vi "hmi_browse_builder_class.vi"(8 "error in (no error)":errorcluster, 11 "project_file":string) -> (0 "error out":errorcluster, 3 "selected path":path)   [LabVIEW 2015, in "lv-build-interface.lvlib"]
uses:
  lv-build-interface.lvlib
  lv-builder/lv-builder.lvlib
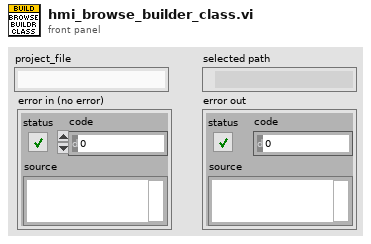
[diagram p1: front panel]
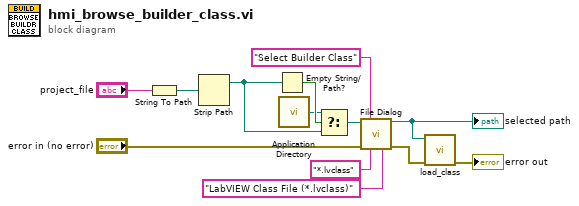
[diagram p0: block diagram]
diagram:
  n1 = String To Path(string="project_file") -> (path=w11:path)
  n2 = Strip Path(path=w11) -> (stripped path=w4:path)  [unwired: 1 out]
  n3 = Empty String/Path?(string/path=w4) -> (empty?=w12:bool)
  n4 = call <vilib>:"Application Directory.vi"() -> ("Application Directory"=w9:path)
  n5 = Select(t=w9, s=w12, f=w4) -> (s? t:f=w13:path)
  n6 = call "File Dialog"("start path"=w13, "prompt"="Select Builder Class", "error in"="error in (no error)", "pattern (all files)"="*.lvclass" ("filter"), "pattern label"="LabVIEW Class File (*.lvclass)" ("filter")) -> ("selected path"=w3:path, "error out"=w2:errorcluster)  [unwired: 7 in, 2 out]
  "selected path" <- w3
  n7 = call "load_class.vi"("error in (no error)"=w2, "class"=w3) -> ("error out"=→"error out":errorcluster)  [unwired: 8 in, 1 out]
